vi "Initialize Instrument.vi"(8 "error in (no error)":errorcluster, 10 "Reset":bool, 11 "Power Supply in":refnum<class "Power Supply.lvclass">) -> (0 "error out":errorcluster, 3 "Power Supply out":refnum<class "Power Supply.lvclass">)   [LabVIEW 2020, in "Power Supply.lvclass"]
uses:
  Power Supply.lvclass
  C:/Sandbox/Git_Sandbox/WiSpry Test Framework source code (LV20)/WiSpry Test Framework/Instruments/Instrument.lvclass
  Instrument.lvclass/Instrument.ctl
  Power Supply.lvclass/Power Supply.ctl
  Instrument.lvclass
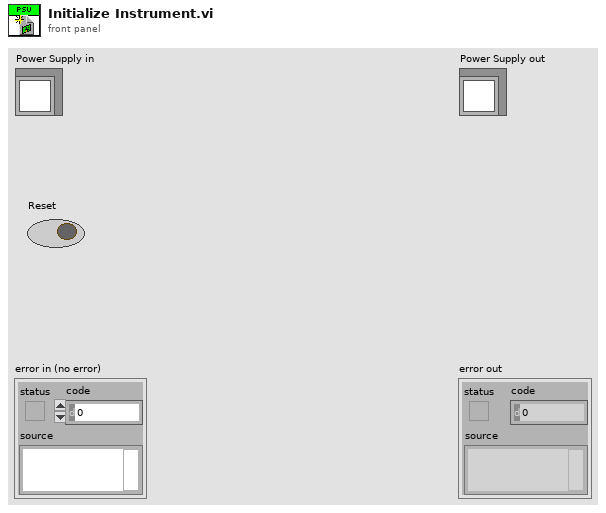
[diagram p1: front panel]
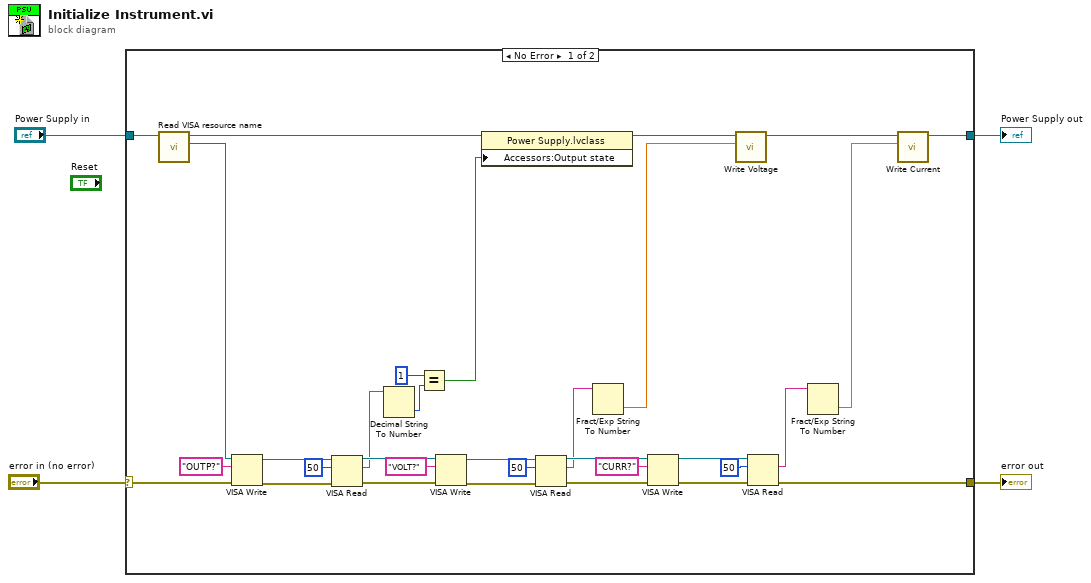
[diagram p0: block diagram]
diagram:
  n1 = case shown="No Error" "error in (no error)" {
    selector: "error in (no error)" -> [w20 w38]
    tunnel: [w19 w38] -> w3
    tunnel: [w11 w37] -> w2
    tunnel: "Power Supply in" -> [w8 w37]
    frame No Error {
      n2 = call "Read VISA resource name.vi"("Instrument in"=w8) -> ("VISA resource name"=w6:refnum<visa-resource-name>, "Instrument out"=w7:refnum<class "Power Supply.lvclass">)  [unwired: 9 in]
      n3 = VISA Write(VISA resource name=w6, write buffer="OUTP?", error in (no error)=w20) -> (VISA resource name out=w36:refnum<visa-resource-name>, error out=w35:errorcluster)  [unwired: 1 out]
      n4 = VISA Read(VISA resource name=w36, byte count=u32 50, error in (no error)=w35) -> (VISA resource name out=w24:refnum<visa-resource-name>, read buffer=w18:string, error out=w23:errorcluster)  [unwired: 1 out]
      n5 = Decimal String To Number(string=w18) -> (number=w17:i32)  [unwired: 2 in, 1 out]
      n6 = Equal?(x=1, y=w17) -> (x = y?=w5:bool)
      n7 = VISA Write(VISA resource name=w24, write buffer="VOLT?", error in (no error)=w23) -> (VISA resource name out=w29:refnum<visa-resource-name>, error out=w30:errorcluster)  [unwired: 1 out]
      n8 = property class="Power Supply.lvclass"(reference=w7, "Accessors:Output state"=w5) -> (reference out=w13:refnum<class "Power Supply.lvclass">)  [unwired: 1 in, 1 out]
      n9 = VISA Read(VISA resource name=w29, byte count=u32 50, error in (no error)=w30) -> (VISA resource name out=w22:refnum<visa-resource-name>, read buffer=w14:string, error out=w21:errorcluster)  [unwired: 1 out]
      n10 = Fract/Exp String To Number(string=w14) -> (number=w10:dbl)  [unwired: 3 in, 1 out]
      n11 = VISA Write(VISA resource name=w22, write buffer="CURR?", error in (no error)=w21) -> (VISA resource name out=w28:refnum<visa-resource-name>, error out=w27:errorcluster)  [unwired: 1 out]
      n12 = call "Write Voltage.vi"("Voltage"=w10, "Power Supply in"=w13) -> ("Power Supply out"=w12:refnum<class "Power Supply.lvclass">)  [unwired: 9 in]
      n13 = VISA Read(VISA resource name=w28, byte count=u32 50, error in (no error)=w27) -> (read buffer=w15:string, error out=w19:errorcluster)  [unwired: 2 out]
      n14 = Fract/Exp String To Number(string=w15) -> (number=w9:dbl)  [unwired: 3 in, 1 out]
      n15 = call "Write Current.vi"("Current"=w9, "Power Supply in"=w12) -> ("Power Supply out"=w11:refnum<class "Power Supply.lvclass">)  [unwired: 9 in]
    }
    frame Error {
    }
  }
  "error out" <- w3
  "Power Supply out" <- w2
